vi "Run or Halt Fan.vi"(8 "error in (no error)":cluster{"状态":bool, "代码":i32, "源":string} caption="错误输入（无错误）", 10 "正在运行？":bool=TRUE, 11 "双风扇输入":refnum<class "Dual Fan.lvclass">) -> (0 "error out":cluster{"状态":bool, "代码":i32, "源":string} caption="错误输出", 3 "双风扇输出":refnum<class "Dual Fan.lvclass">)   [LabVIEW 2013, in "Dual Fan.lvlib" / "Dual Fan.lvclass"]
doc: "调用该方法以通知风扇启动或停止运行。"
uses:
  Dual Fan.lvclass
  Dual Fan.lvclass/Dual Fan.ctl
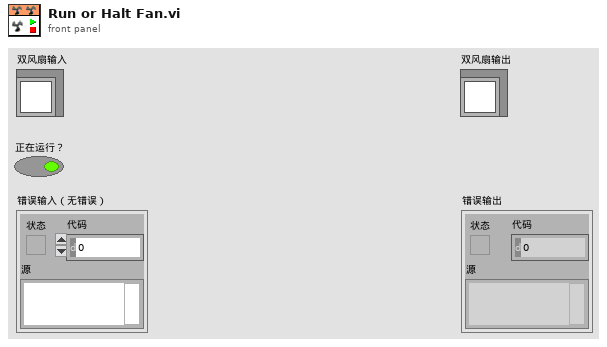
[diagram p1: front panel]
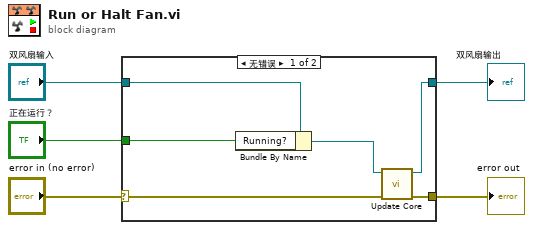
[diagram p0: block diagram]
diagram:
  n1 = case shown="无错误" "error in (no error)" {
    selector: "error in (no error)" -> [w7 w13]
    tunnel: [w8 w13] -> w4
    tunnel: [w9 w12] -> w2
    tunnel: "双风扇输入" -> [w11 w12]
    tunnel: "正在运行？" -> [w6 _]
    frame No Error {
      n2 = Bundle By Name(cluster=w11, "Running?"=w6) -> (w10:refnum<class "Dual Fan.lvclass">)
      n3 = call-dynamic "Update Core.vi"("error in (no error)"=w7, "双风扇输入"=w10) -> ("error out"=w8:cluster{"状态":bool, "代码":i32, "源":string}, "双风扇输出"=w9:refnum<class "Dual Fan.lvclass">)  [unwired: 8 in]
    }
    frame Error {
    }
  }
  "error out" <- w4
  "双风扇输出" <- w2
